vi "Send Current Grabber State.vi"(7 "Message Priority (Normal)":T2=enum."Normal", 8 "error in (no error)":errorcluster, 9 "Grabber.lvlib:Current Grabber State Msg.lvclass":refnum<class "Current Grabber State Msg.lvclass">, 10 "Grabber State":T1, 11 "Message Enqueuer":refnum<class "Message Enqueuer.lvclass">) -> (0 "error out":errorcluster, 3 "Message Enqueuer out":refnum<class "Message Enqueuer.lvclass">)   [LabVIEW 2014, in "Grabber.lvlib" / "Current Grabber State Msg.lvclass"]
doc: "This VI sends the message to an actor."
uses:
  Current Grabber State Msg.lvclass
  <vilib>/ActorFramework/Message Enqueuer/Message Enqueuer.lvclass
  <vilib>/ActorFramework/Message Enqueuer/Message Priority.ctl
  Grabber Class/Grabber State.ctl
  Current Grabber State Msg.lvclass/Current Grabber State Msg.ctl
  <vilib>/ActorFramework/Message Enqueuer/Message Enqueuer.lvclass/Message Enqueuer.ctl
  <vilib>/ActorFramework/Message Priority Queue/Priority Enqueue.vi
  Grabber Class/Grabber.lvclass
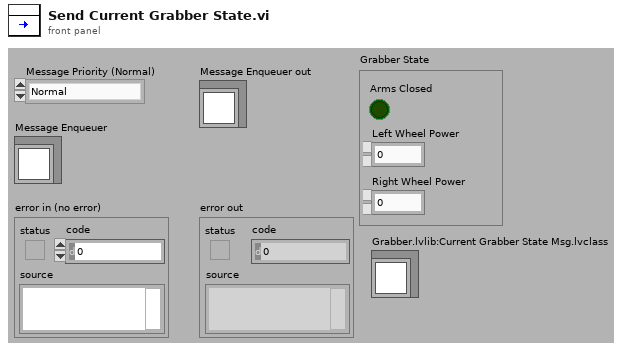
[diagram p1: front panel]
types:
  T1 = typedef "Grabber.lvlib/Grabber.lvclass/Grabber State.ctl" = cluster{"Arms Closed":bool, "Left Wheel Power":dbl, "Right Wheel Power":dbl}
  T2 = typedef "Actor Framework.lvlib/Message Enqueuer.lvclass/Message Priority.ctl" = enum16{"Low", "Normal", "High"}
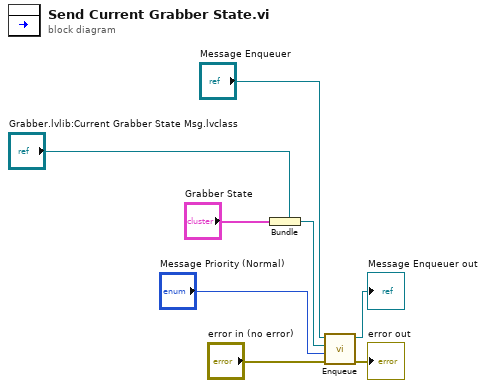
[diagram p0: block diagram]
diagram:
  n1 = Bundle(cluster="Grabber.lvlib:Current Grabber State Msg.lvclass", "Grabber State") -> (w2:refnum<class "Current Grabber State Msg.lvclass">)
  n2 = call <vilib>:"Enqueue.vi"("error in (no error)"="error in (no error)", "Message Priority (Normal)"="Message Priority (Normal)", "Message"=w2, "Message Enqueuer in"="Message Enqueuer") -> ("error out"=→"error out":errorcluster, "Message Enqueuer out"=→"Message Enqueuer out":refnum<class "Message Enqueuer.lvclass">)  [unwired: 6 in]
